vi "Serial Output Channel Datapath.vi"(0 "start trigger":bool, 1 "reset":bool, 2 "resources":T13, 5 "stop trigger":bool, 7 "generation counter":T11, 9 "output valid":bool, 11 "tagged llp packet":T2, 12 "configuration":T19, 13 "dram status":T1) -> (4 "channel status":T12, 10 "ready for start trigger":bool, 14 "ready for input":bool)   [LabVIEW 2020, in "GettingStarted_Gen_148X_FPGA.lvlib"]
uses:
  GettingStarted_Gen_148X_FPGA.lvlib
  Types/Serial Output Channel Datapath Configuration.ctl
  Types/Serial Output Channel Resources.ctl
  Common/Types/Serial Output Channel IO.ctl
  Common/Types/Serial Output Channel IO 32b.ctl
  Common/Types/Serial Output Channel IO 64b.ctl
  Common/Types/I2C IO.ctl
  Common/Types/Single Serial Channel Resources.ctl
  Types/Serial Output Channel Status.ctl
  Common/Types/DRAM Status.ctl
  <instrlib>/FlexRIO/CSI-2/v2/FPGA/Types/Timestamp Counter Value.ctl
  <instrlib>/FlexRIO/CSI-2/v2/FPGA/Types/Tagged LLP Packet.ctl
  <instrlib>/FlexRIO/CSI-2/v2/FPGA/Types/FPGA LLP Packet Tag.ctl
  <instrlib>/FlexRIO/CSI-2/v2/FPGA/Types/FPGA LLP Packet Timestamp.ctl
  <instrlib>/FlexRIO/CSI-2/v2/FPGA/Types/Timestamp ID.ctl
  <instrlib>/FlexRIO/CSI-2/v2/FPGA/Types/FPGA LLP Packet Size.ctl
  <instrlib>/FlexRIO/CSI-2/v2/FPGA/Types/LLP Packet.ctl
  <instrlib>/FlexRIO/CSI-2/v2/FPGA/Types/LLP Packet Header.ctl
  <instrlib>/FlexRIO/CSI-2/v2/FPGA/Types/LLP Packet Payload.ctl
  <instrlib>/FlexRIO/CSI-2/v2/FPGA/Types/LLP Packet Footer.ctl
  Common/GettingStarted_Common_148X_FPGA.lvlib
  <instrlib>/FlexRIO/CSI-2/v2/FPGA/NI CSI-2 API FPGA v2.lvlib
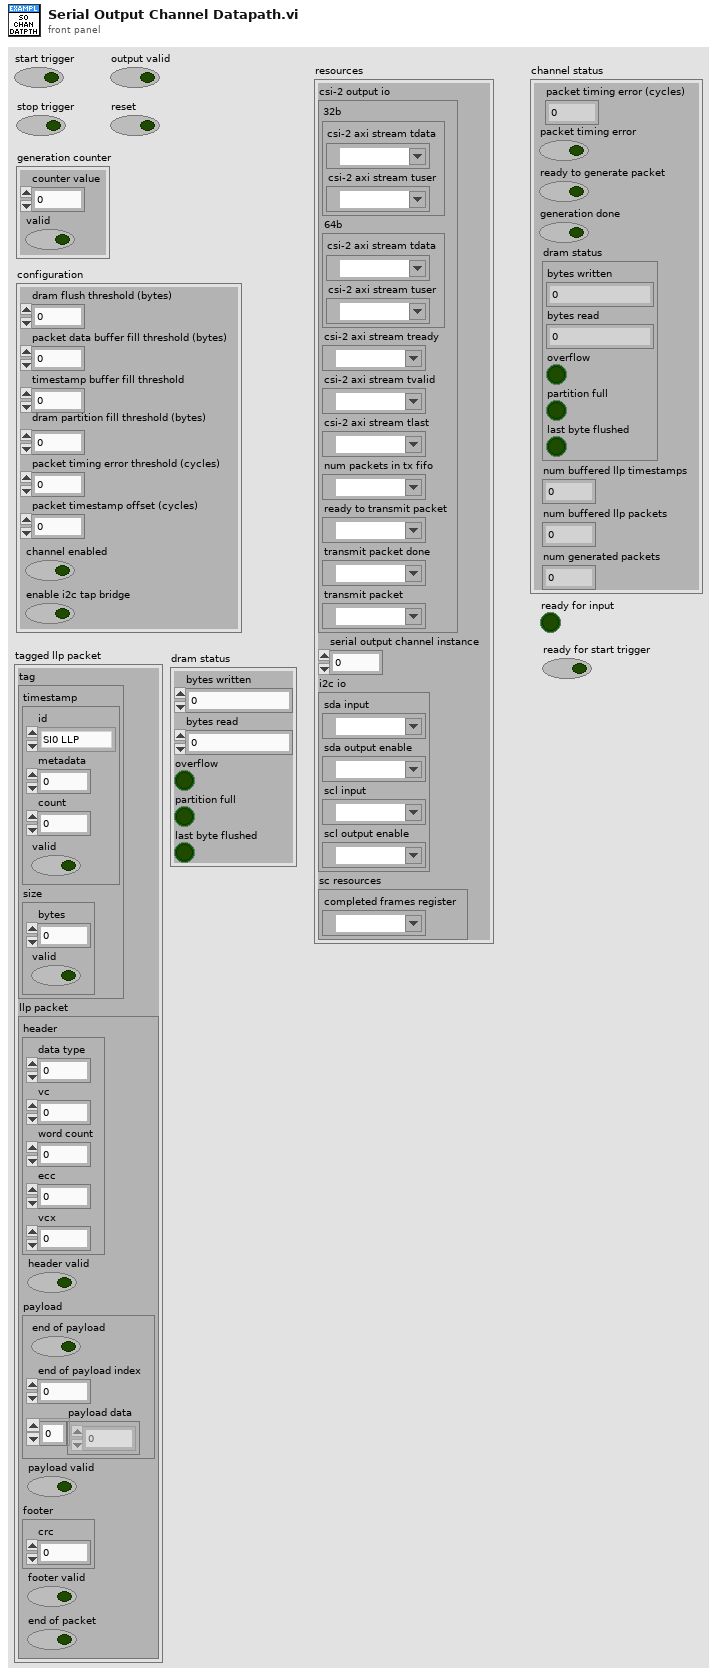
[diagram p1: front panel]
types:
  T1 = typedef "GettingStarted_Common_148X_FPGA.lvlib/DRAM Status.ctl" = cluster{"bytes written":u64, "bytes read":u64, "overflow":bool, "partition full":bool, "last byte flushed":bool}
  T2 = typedef "NI CSI-2 API FPGA v2.lvlib/Tagged LLP Packet.ctl" = cluster{"tag":T3, "llp packet":T7}
  T3 = typedef "NI CSI-2 API FPGA v2.lvlib/FPGA LLP Packet Tag.ctl" = cluster{"timestamp":T4, "size":T6}
  T4 = typedef "NI CSI-2 API FPGA v2.lvlib/FPGA LLP Packet Timestamp.ctl" = cluster{"valid":bool, "count":fxp<+,50,50>, "id":T5, "metadata":u8}
  T5 = typedef "NI CSI-2 API FPGA v2.lvlib/Timestamp ID.ctl" = enum8{"SI0 LLP", "SI1 LLP", "SI2 LLP", "SI3 LLP", "SI4 LLP", "SI5 LLP", "SI6 LLP", "SI7 LLP", "SO0 LLP", "SO1 LLP", "SO2 LLP", "SO3 LLP", "SO4 LLP", "SO5 LLP", "SO6 LLP", "SO7 LLP", "Ser0 GPIO Bank", "Ser1 GPIO Bank", "Ser2 GPIO Bank", "Ser3 GPIO Bank", "Ser4 GPIO Bank", "Ser5 GPIO Bank", "Ser6 GPIO Bank", "Ser7 GPIO Bank", "Des0 GPIO Bank", "Des1 GPIO Bank", "Des2 GPIO Bank", "Des3 GPIO Bank", "Des4 GPIO Bank", "Des5 GPIO Bank", "Des6 GPIO Bank", "Des7 GPIO Bank", "User0", "User1", "User2", "User3", "User4", "User5", "User6", "User7", "User8", "User9", "User10", "User11", "User12", "User13", "User14", "User15", "User16", "User17", "User18", "User19", "User20", "User21", "User22", "User23", "User24", "User25", "User26", "User27", "User28", "User29", "User30", "User31"}
  T6 = typedef "NI CSI-2 API FPGA v2.lvlib/FPGA LLP Packet Size.ctl" = cluster{"bytes":fxp<+,17,17>, "valid":bool}
  T7 = typedef "NI CSI-2 API FPGA v2.lvlib/LLP Packet.ctl" = cluster{"header":T8, "header valid":bool, "payload":T9, "payload valid":bool, "footer":T10, "footer valid":bool, "end of packet":bool}
  T8 = typedef "NI CSI-2 API FPGA v2.lvlib/LLP Packet Header.ctl" = cluster{"word count":u16, "ecc":fxp<+,6,6>, "vcx":fxp<+,2,2>, "data type":fxp<+,6,6>, "vc":fxp<+,2,2>}
  T9 = typedef "NI CSI-2 API FPGA v2.lvlib/LLP Packet Payload.ctl" = cluster{"end of payload":bool, "end of payload index":fxp<+,3,3>, "payload data":u8[]}
  T10 = typedef "NI CSI-2 API FPGA v2.lvlib/LLP Packet Footer.ctl" = cluster{"crc":u16}
  T11 = typedef "NI CSI-2 API FPGA v2.lvlib/Timestamp Counter Value.ctl" = cluster{"counter value":u64, "valid":bool}
  T12 = typedef "GettingStarted_Gen_148X_FPGA.lvlib/Serial Output Channel Status.ctl" = cluster{"num buffered llp packets":fxp<+,14,14>, "packet timing error (cycles)":u64, "packet timing error":bool, "ready to generate packet":bool, "dram status":T1, "num buffered llp timestamps":u32, "generation done":bool, "num generated packets":u64}
  T13 = typedef "GettingStarted_Gen_148X_FPGA.lvlib/Serial Output Channel Resources.ctl" = cluster{"csi-2 output io":T14, "serial output channel instance":u8, "i2c io":T17, "sc resources":T18}
  T14 = typedef "GettingStarted_Common_148X_FPGA.lvlib/Serial Output Channel IO.ctl" = cluster{"32b":T15, "64b":T16, "csi-2 axi stream tready":refnum<k21>, "csi-2 axi stream tvalid":refnum<k21>, "csi-2 axi stream tlast":refnum<k21>, "num packets in tx fifo":refnum<k21>, "ready to transmit packet":refnum<k21>, "transmit packet done":refnum<k21>, "transmit packet":refnum<k21>}
  T15 = typedef "GettingStarted_Common_148X_FPGA.lvlib/Serial Output Channel IO 32b.ctl" = cluster{"csi-2 axi stream tdata":refnum<k21>, "csi-2 axi stream tuser":refnum<k21>}
  T16 = typedef "GettingStarted_Common_148X_FPGA.lvlib/Serial Output Channel IO 64b.ctl" = cluster{"csi-2 axi stream tdata":refnum<k21>, "csi-2 axi stream tuser":refnum<k21>}
  T17 = typedef "GettingStarted_Common_148X_FPGA.lvlib/I2C IO.ctl" = cluster{"sda input":refnum<k21>, "sda output enable":refnum<k21>, "scl input":refnum<k21>, "scl output enable":refnum<k21>}
  T18 = typedef "GettingStarted_Common_148X_FPGA.lvlib/Single Serial Channel Resources.ctl" = cluster{"completed frames register":refnum<k21>}
  T19 = typedef "GettingStarted_Gen_148X_FPGA.lvlib/Serial Output Channel Datapath Configuration.ctl" = cluster{"dram flush threshold (bytes)":u64, "packet data buffer fill threshold (bytes)":u64, "timestamp buffer fill threshold":u32, "packet timing error threshold (cycles)":u64, "channel enabled":bool, "dram partition fill threshold (bytes)":u64, "enable i2c tap bridge":bool, "packet timestamp offset (cycles)":i64}
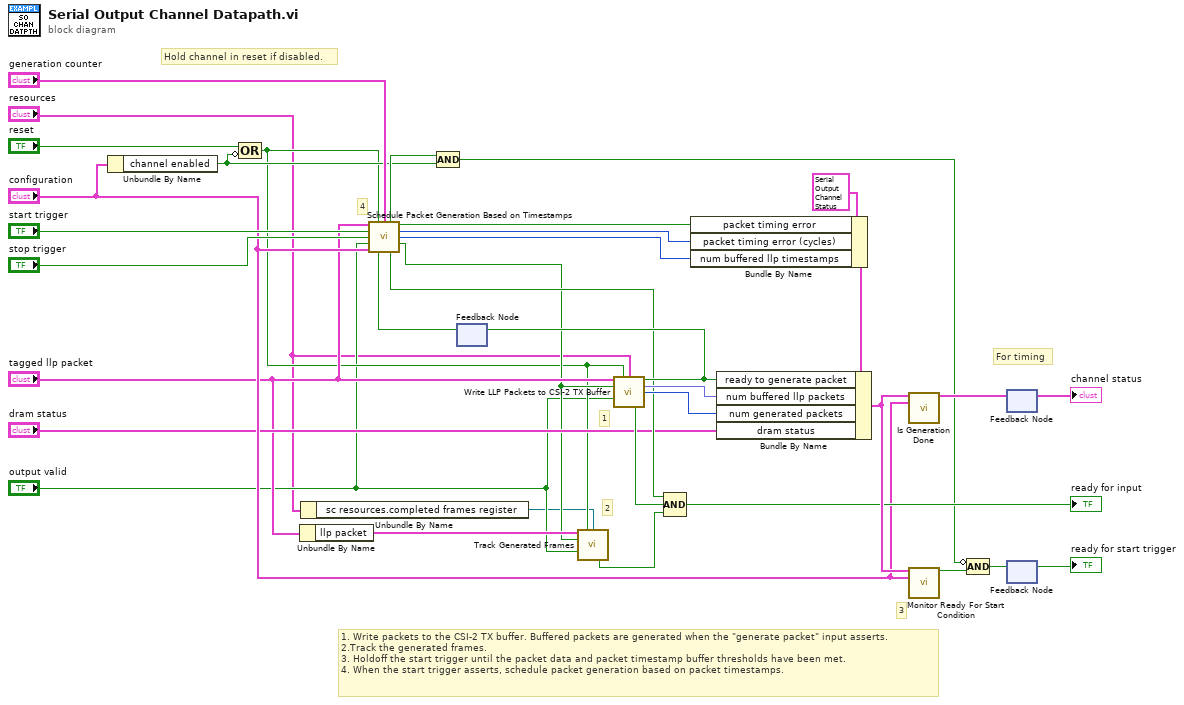
[diagram p0: block diagram]
diagram:
  # "2"
  # "3"
  # "4"
  # "1"
  # "1. Write packets to the CSI-2 TX buffer. Buffered packets are generated when the \"generate packet\" input asserts.\n2.Track the generated frames.\n3. Holdoff the start trigger until the packet data and packet timestamp buffer thresholds have been met.\n4. When the start trigger asserts, schedule packet generation based on packet timestamps."
  # "Hold channel in reset if disabled."
  # "For timing"
  n1 = Unbundle By Name("configuration") -> ("channel enabled"=w11:bool)
  n2 = Compound Arithmetic op=OR("reset", invert w11) -> (w5:bool)
  n3 = Unbundle By Name("tagged llp packet") -> ("llp packet"=w8:T7)
  n4 = Unbundle By Name("resources") -> ("sc resources.completed frames register"=w1:refnum<k21>)
  n5 = feedback #1() -> (w30:bool)  [unwired: 1 in]
  n6 = call "Schedule Packet Generation Based on Timestamps.vi"("tagged llp packet"="tagged llp packet", "reset"=w5, "generation counter"="generation counter", "start trigger"="start trigger", "stop trigger"="stop trigger", "tagged llp packet valid"="output valid", "configuration"="configuration", "ready to generate packet"=w30) -> ("in reset"=w12:bool, "packet timing error"=w29:bool, "packet timing error (cycles)"=w28:u64, "number of buffered llp timestamps"=w27:u32, "generate packet"=w7:bool, "ready for tagged llp packet"=w14:bool)  [unwired: 2 in]
  n7 = Compound Arithmetic op=AND(w12, w11) -> (w6:bool)
  n8 = call "Track Generated Frames.vi"("llp packet"=w8, "reset"=w5, "completed frames register"=w1, "generate packet"=w7, "input valid"="output valid") -> ("ready for input"=w3:bool)  [unwired: 10 in]
  n9 = call "Write LLP Packets to CSI-2 TX Buffer.vi"("tagged llp packet"="tagged llp packet", "reset"=w5, "resources"="resources", "generate packet"=w7, "input valid"="output valid") -> ("ready to generate packet"=w18:bool, "num packets in tx buffer"=w31:fxp<+,14,14>, "num generated packets"=w21:u64, "ready for input"=w20:bool)  [unwired: 7 in]
  n10 = feedback-in #1(w18) -> ()
  n11 = Compound Arithmetic op=AND(w14, w20, w3) -> (→"ready for input":bool)
  n12 = Bundle By Name(cluster=T12 {"num buffered llp packets"=0.0, "packet timing error (cycles)"=0, "packet timing error"=FALSE, "ready to generate packet"=FALSE, "dram status"={"bytes written"=0, "bytes read"=0, "overflow"=FALSE, "partition full"=FALSE, "last byte flushed"=FALSE}, "num buffered llp timestamps"=0, "generation done"=FALSE, "num generated packets"=0}, "packet timing error"=w29, "packet timing error (cycles)"=w28, "num buffered llp timestamps"=w27) -> (w33:T12)
  n13 = Bundle By Name(cluster=w33, "ready to generate packet"=w18, "num buffered llp packets"=w31, "num generated packets"=w21, "dram status"="dram status") -> (w23:T12)
  n14 = call "Is Generation Done.vi"("channel status in"=w23, "configuration"="configuration") -> ("channel status out"=w22:T12)  [unwired: 13 in]
  n15 = call "Monitor Ready For Start Condition.vi"("channel status"=w23, "configuration"="configuration") -> ("ready for start"=w24:bool)  [unwired: 13 in]
  n16 = Compound Arithmetic op=AND(invert w6, w24) -> (w13:bool)
  n17 = feedback-in #2(w22) -> ()
  n18 = feedback #2() -> (→"channel status":T12)  [unwired: 1 in]
  n19 = feedback #3() -> (→"ready for start trigger":bool)  [unwired: 1 in]
  n20 = feedback-in #3(w13) -> ()
